vi "Configure.vi"(8 "error in (no error)":errorcluster, 11 "Piezo in":refnum<class "Piezo.lvclass">) -> (0 "error out":errorcluster, 2 "cancelled?":bool, 3 "Piezo out":refnum<class "Piezo.lvclass">)   [LabVIEW 2012, in "Piezo.lvclass"]
doc: "The configure method configures the details for the RabbitMQ connection, the observers and the mapping script.\n\nIn the derived class, make a call to the parent for setting these parameters."
uses:
  Piezo.lvclass
  <vilib>/Utility/miscctls.llb/LVPointTypeDef.ctl
  Piezo.lvclass/Piezo.ctl
  <vilib>/Distrio/Murmex/Murmex/Murmex.lvclass
panel:
  in  "button:call parent":bool
  in  "button:ok":bool
  in  "button:cancel":bool
  in  "Tab Control":enum32{"Task"}(tab)
  in  "Reporting folder":path
  in  "Micron to voltage\nconversion factor":dbl[unit]
  in  "Min V":dbl
  in  "Max V":dbl
  in  "Analog output":tag
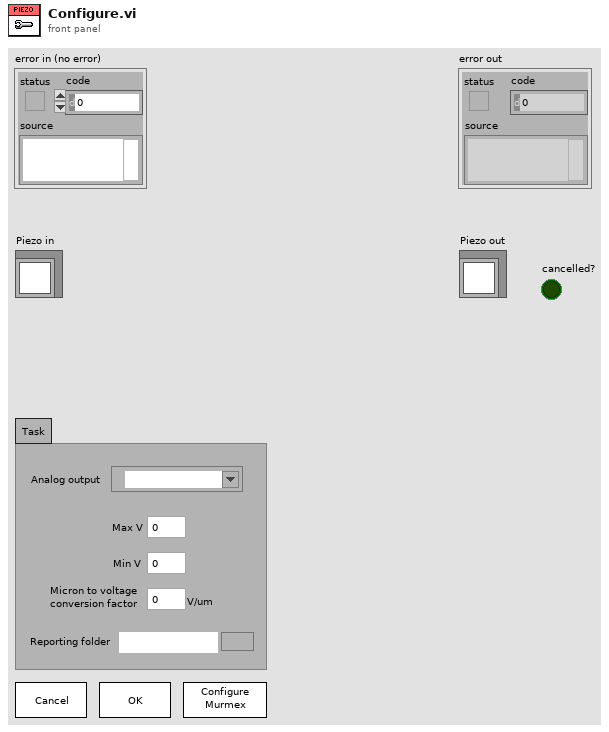
[diagram p1: front panel]
types:
  T1 = typedef "LVPointTypeDef.ctl" = cluster{"Horizontal":i16, "Vertical":i16}
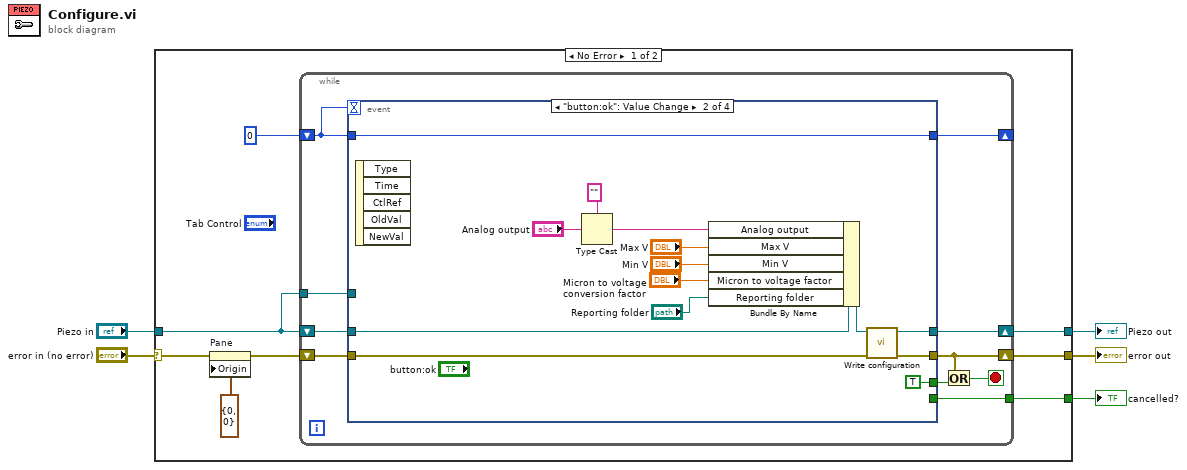
[diagram p0: block diagram]
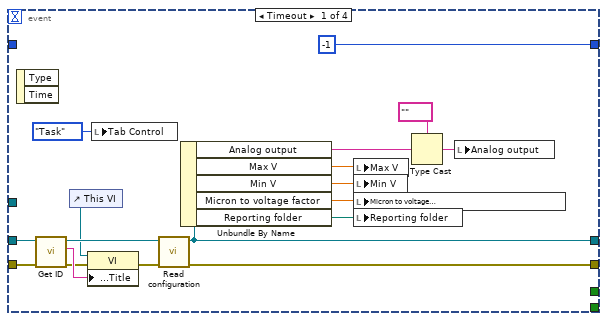
[diagram p2: hidden frame]
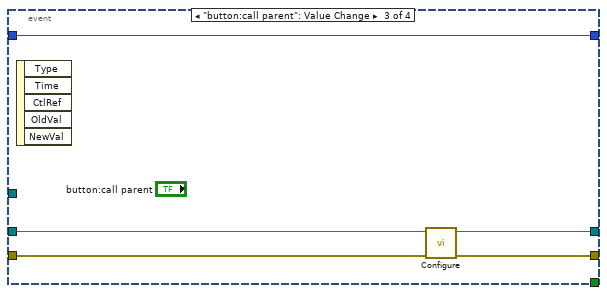
[diagram p3: hidden frame]
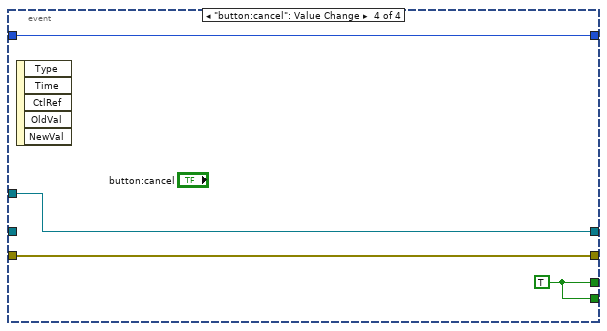
[diagram p4: hidden frame]
diagram:
  n1 = case shown="No Error" "error in (no error)" {
    selector: "error in (no error)" -> [w12 w66]
    tunnel: "Piezo in" -> [w10 w65]
    tunnel: [w7 w66] -> w3
    tunnel: [w8 w65] -> w2
    tunnel: [w6 _] -> w1
    frame No Error {
      n2 = property on="Pane" class="Pane"(error in=w12, "Origin"=T1 {"Horizontal"=0, "Vertical"=0}) -> (error out=w11:errorcluster)  [unwired: 1 in, 1 out]
      n3 = while {
        shift-right: [w17] -> w7
        shift-left: w11 -> [w21]
        shift-right: [w19] -> w8
        shift-left: w10 -> [w20]
        tunnel: w10 -> [w18]
        shift-right: [w22] -> _
        shift-left: 0 -> [w23]
        tunnel: [w14] -> w6
        stop <- w16 stop-if-true
        n4 = event shown="[1] \"button:ok\": Value Change" {
          selector: _ -> [_ _ _ _]
          dyn-events: _ -> [_ _ _ _]
          timeout: w23 -> [_ _ _ _]
          tunnel: w23 -> [_ w45 w56 w62]
          tunnel: [-1 w45 w56 w62] -> w22
          tunnel: w21 -> [w34 w53 w60 w63]
          tunnel: [w33 w55 w59 w63] -> w17
          tunnel: w20 -> [w32 w52 w57 _]
          tunnel: [w31 w54 w58 w64] -> w19
          tunnel: w18 -> [_ _ _ w64]
          tunnel: [_ TRUE _ w61] -> w15
          tunnel: [_ _ _ w61] -> w14
          event Timeout {
            n5 = event-data() -> ()  [unwired: 1 in, 2 out]
            n6 = call <vilib>:"Get ID.vi"("error in (no error)"=w34, "Murmex in"=w32) -> ("error out"=w35:errorcluster, "component id"=w39:string, "Murmex out"=w38:refnum<class "Piezo.lvclass">)  [unwired: 7 in]
            n7 = control-ref of="This VI"() -> (w36:refnum<vi>)
            n8 = property class="VI"(reference=w36, error in=w35, "Front Panel.Title"=w39) -> (error out=w37:errorcluster)  [unwired: 1 out]
            n9 = local write "Tab Control"(enum32{"Task"}."Task" ("Tab Control")) -> ()
            n10 = call <vilib>:"Read configuration.vi"("error in (no error)"=w37, "Murmex in"=w38) -> ("error out"=w33:errorcluster, "Murmex out"=w31:refnum<class "Piezo.lvclass">)  [unwired: 7 in, 1 out]
            n11 = Unbundle By Name(w31) -> ("Analog output"=w27:string, "Max V"=w30:dbl, "Min V"=w29:dbl, "Micron to voltage factor"=w28:dbl[unit], "Reporting folder"=w24:path)
            n12 = local write "Max V"(w30) -> ()
            n13 = local write "Min V"(w29) -> ()
            n14 = local write "Micron to voltage\nconversion factor"(w28) -> ()
            n15 = local write "Reporting folder"(w24) -> ()
            n16 = Type Cast(type=tag "" ("Analog output"), x=w27) -> (*(type *) &x=w25:tag)
            n17 = local write "Analog output"(w25) -> ()
          }
          event "button:ok": Value Change {
            n18 = event-data() -> ()  [unwired: 1 in, 5 out]
            n19 = Type Cast(type="" ("configuration.Analog output"), x="Analog output") -> (*(type *) &x=w48:string)
            n20 = Bundle By Name(cluster=w52, "Analog output"=w48, "Max V"="Max V", "Min V"="Min V", "Micron to voltage factor"="Micron to voltage\nconversion factor", "Reporting folder"="Reporting folder") -> (w51:refnum<class "Piezo.lvclass">)
            n21 = call <vilib>:"Write configuration.vi"("error in (no error)"=w53, "Murmex in"=w51) -> ("error out"=w55:errorcluster, "Murmex out"=w54:refnum<class "Piezo.lvclass">)  [unwired: 8 in]
          }
          event "button:call parent": Value Change {
            n22 = event-data() -> ()  [unwired: 1 in, 5 out]
            n23 = call-parent "Configure.vi"("error in (no error)"=w60, "Murmex in"=w57) -> ("error out"=w59:errorcluster, "Murmex out"=w58:refnum<class "Piezo.lvclass">)  [unwired: 7 in, 1 out]
          }
          event "button:cancel": Value Change {
            w61 = TRUE
            n24 = event-data() -> ()  [unwired: 1 in, 5 out]
          }
        }
        n25 = Or(x=w17, y=w15) -> (x .or. y?=w16:bool)
      }
    }
    frame Error {
    }
  }
  "error out" <- w3
  "Piezo out" <- w2
  "cancelled?" <- w1
